vi "Change X Direction.vi"(1 "Vertical Segments Parameters in":T1(array[cluster])) -> (0 "Vertical Segments Parameters out":T1(array[cluster]))   [LabVIEW 2017]
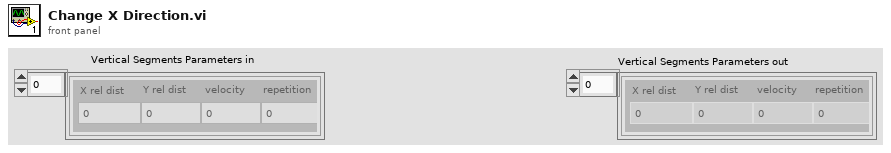
[diagram p1: front panel]
types:
  T1 = cluster{"X rel dist":dbl, "Y rel dist":dbl, "velocity":dbl, "repetition":u32}[]
  T2 = cluster{"X rel dist":i32, "velocity":i32, "rep":i32, "Y rel dist":i32}
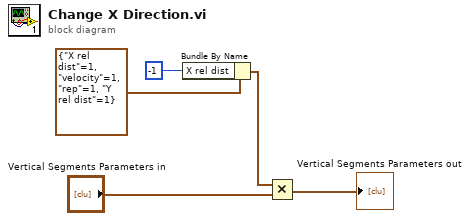
[diagram p0: block diagram]
diagram:
  n1 = Bundle By Name(cluster=T2 {"X rel dist"=1, "velocity"=1, "rep"=1, "Y rel dist"=1} ("Vertical Segments Parameters"), "X rel dist"=-1 ("X factor")) -> (w1:T2)
  n2 = Multiply(x=w1, y="Vertical Segments Parameters in") -> (x*y=→"Vertical Segments Parameters out":cluster{"X rel dist":dbl, dbl, dbl, u32}[])
